vi "Create Actual Array.vi"(1 "Boolean array":bool[](array[boolean])=[FALSE, FALSE, FALSE, FALSE, FALSE, FALSE, FALSE, FALSE]) -> (0 "Ouptut Array":bool[](array[boolean]))   [LabVIEW 2017]
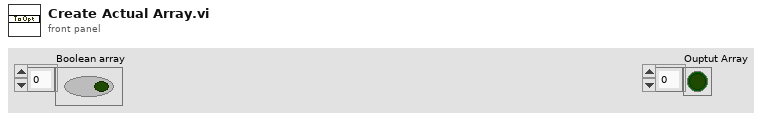
[diagram p1: front panel]
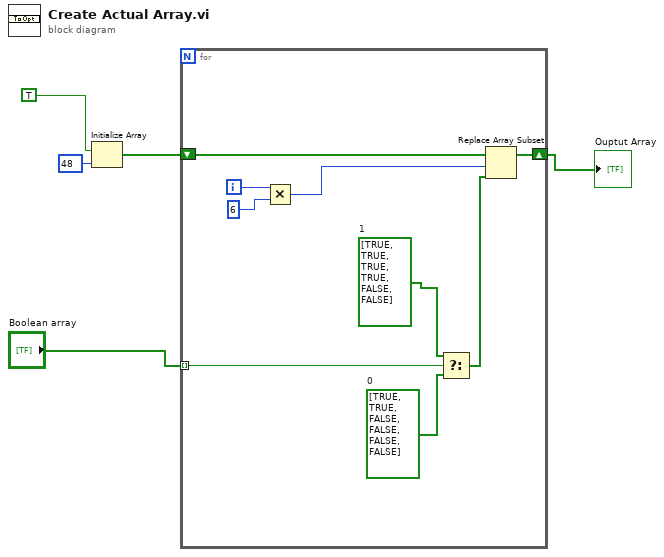
[diagram p0: block diagram]
diagram:
  n1 = Initialize Array(TRUE, 48 ("dimension size")) -> (w3:bool[])
  n2 = for {
    tunnel: "Boolean array" -> [w14] mode=indexing
    shift-right: [w6] -> w1
    shift-left: w3 -> [w11]
    i -> [w10]
    w13 = bool[] [TRUE, TRUE, TRUE, TRUE, FALSE, FALSE]  # 1
    w12 = bool[] [TRUE, TRUE, FALSE, FALSE, FALSE, FALSE]  # 0
    n3 = Multiply(x=w10, y=6) -> (x*y=w8:i32)
    n4 = Select(t=w13, s=w14, f=w12) -> (s? t:f=w7:bool[])
    n5 = Replace Array Subset(array=w11, new element=w7, index=w8) -> (w6:bool[])
  }
  "Ouptut Array" <- w1
